vi "Actor Core.vi"(8 "error in":errorcluster, 11 "Hardware in":refnum<class "thorlabs_panel.lvclass">) -> (0 "error out":errorcluster, 3 "Actor out":refnum<class "Actor.lvclass">)   [LabVIEW 2015, in "thorlabs_panel.lvclass"]
doc: "(<B>Filename</B>: Actor Framework.lvlib:Actor.lvclass:Actor Core.vi)\n\nReceives messages to the actor, reacts to them, and initiates any error handling that may shut the actor down.\n\nDescendant classes may override this VI to append parallel tasks for the actor to complete while it handles messages. Overrides use the Call Parent Method node."
uses:
  thorlabs_panel.lvclass
  <vilib>/ActorFramework/Actor/Actor.lvclass
  UI/panel_class/panel.lvclass/panel.ctl
  <vilib>/ActorFramework/Actor/Actor.lvclass/Actor.ctl
  <vilib>/ActorFramework/Message Enqueuer/Message Enqueuer.lvclass/Message Enqueuer.ctl
  thorlabs_panel Messages/thorlabs_move_piezos Msg/thorlabs_move_piezos Msg.lvclass/thorlabs_move_piezos Msg.ctl
  thorlabs_panel Messages/thorlabs_connect Msg/thorlabs_connect Msg.lvclass/thorlabs_connect Msg.ctl
  <vilib>/ActorFramework/Message Enqueuer/Init from Existing Queue.vi
  <vilib>/ActorFramework/Message Enqueuer/Enqueue.vi
  <vilib>/ActorFramework/Message Priority Queue/Priority Enqueue.vi
  <vilib>/ActorFramework/Message Enqueuer/Message Enqueuer.lvclass
  thorlabs_panel Messages/thorlabs_move_piezos Msg/thorlabs_move_piezos Msg.lvclass
  thorlabs_panel Messages/thorlabs_zero_piezos Msg/thorlabs_zero_piezos Msg.lvclass
  thorlabs_panel Messages/thorlabs_connect Msg/thorlabs_connect Msg.lvclass
  thorlabs_panel Messages/thorlabs_query_positions Msg/thorlabs_query_positions Msg.lvclass
  UI/panel_class/panel.lvclass
panel:
  in  "step":dbl
  in  "right":bool
  in  "left":bool
  in  "down":bool
  in  "up":bool
  in  "zero_piezos":bool
  out "Z":dbl
  out "Y":dbl
  out "X":dbl
  in  "Speed":dbl
  in  "move_kinesis":bool
  in  "Z":dbl
  in  "Y":dbl
  in  "X":dbl
  out "Status":string
  in  "connect_kinesis":bool
  in  "Controller Serial":string="71827519"
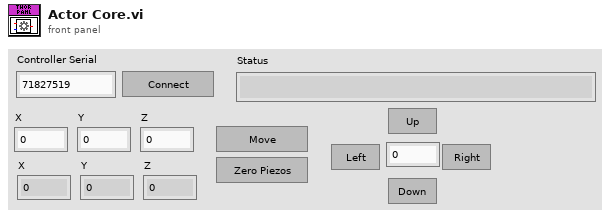
[diagram p1: front panel]
types:
  T1 = typedef "thorlabs_event_refs.ctl" = cluster{"Event Registration Refnum":refnum<event-registration>, "Event Registration Refnum":refnum<event-registration>}
  T2 = cluster{"Event Registration Refnum":refnum<event-registration>, "stop_ui_ref":refnum<event-registration>, "Event Registration Refnum":refnum<event-registration>}
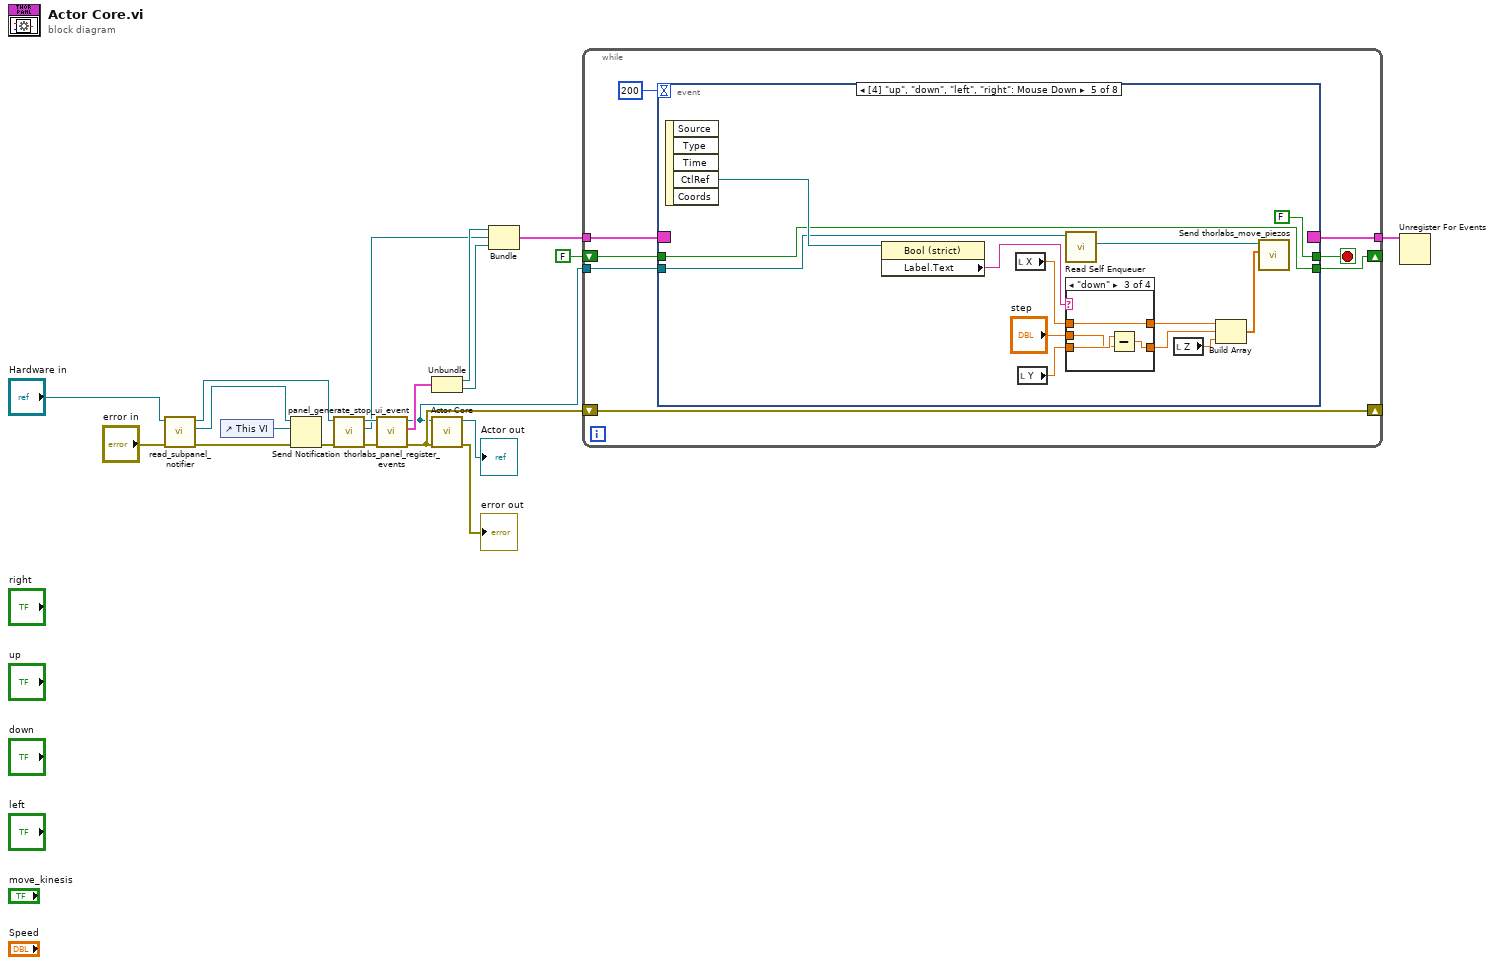
[diagram p0: block diagram]
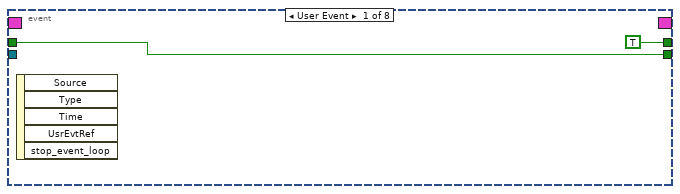
[diagram p2: hidden frame]
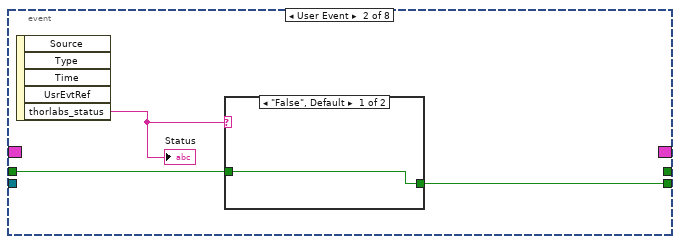
[diagram p3: hidden frame]
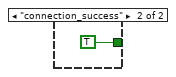
[diagram p4: hidden frame]
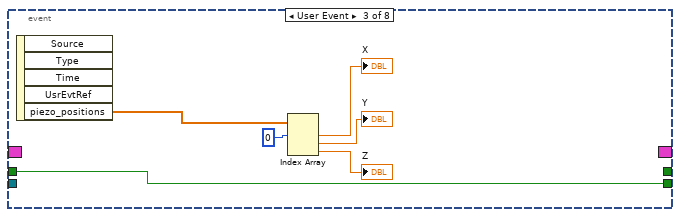
[diagram p5: hidden frame]
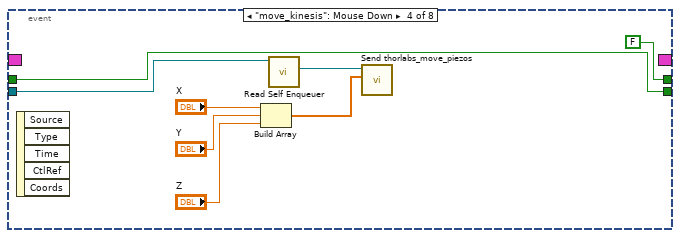
[diagram p6: hidden frame]
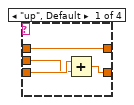
[diagram p7: hidden frame]
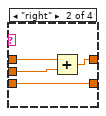
[diagram p8: hidden frame]
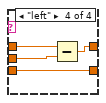
[diagram p9: hidden frame]
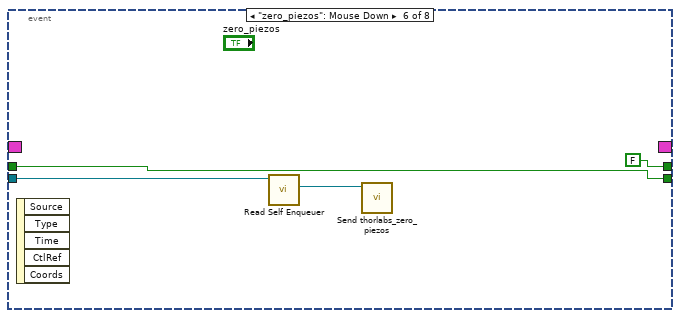
[diagram p10: hidden frame]
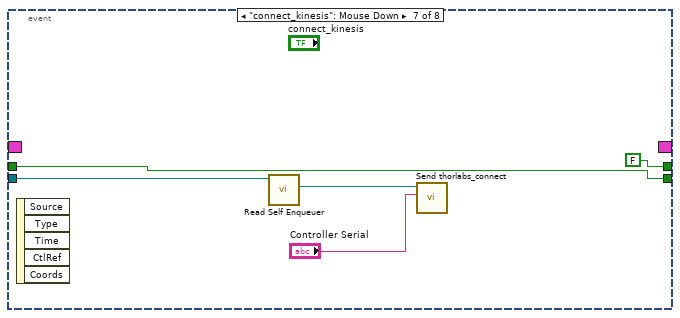
[diagram p11: hidden frame]
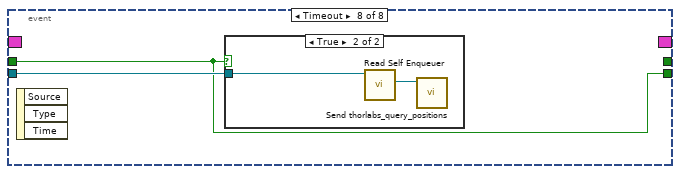
[diagram p12: hidden frame]
diagram:
  n1 = call "read_subpanel_notifier.vi"("error in (no error)"="error in", "panel in"="Hardware in") -> ("error out"=w14:errorcluster, "subpanel_notifier"=w16:refnum<notifier>, "panel out"=w15:refnum<class "thorlabs_panel.lvclass">)  [unwired: 7 in]
  n2 = control-ref of="This VI"() -> (w18:refnum<vi>)
  n3 = Send Notification(notification=w18, notifier=w16, error in (no error)=w14) -> (error out=w13:errorcluster)  [unwired: 1 out]
  n4 = call "panel_generate_stop_ui_event.vi"("error in (no error)"=w13, "panel in"=w15) -> ("error out"=w9:errorcluster, "stop_ui_ref"=w5:refnum<event-registration>, "panel out"=w10:refnum<class "thorlabs_panel.lvclass">)  [unwired: 7 in]
  n5 = call "thorlabs_panel_register_events.vi"("error in (no error)"=w9, "thorlabs_panel in"=w10) -> ("error out"=w8:errorcluster, "event_refs cluster"=w7:T1, "thorlabs_panel out"=w2:refnum<class "thorlabs_panel.lvclass">)  [unwired: 7 in]
  n6 = Unbundle(w7) -> ("Event Registration Refnum"=w6:refnum<event-registration>, "Event Registration Refnum"=w4:refnum<event-registration>)
  n7 = call-parent "Actor Core.vi"("error in"=w8, "Actor in"=w2) -> ("error out"=→"error out":errorcluster, "Actor out"=→"Actor out":refnum<class "Actor.lvclass">)  [unwired: 8 in]
  n8 = Bundle("Event Registration Refnum"=w6, "stop_ui_ref"=w5, "Event Registration Refnum"=w4) -> (w3:T2)  [unwired: 1 in]
  n9 = while {
    tunnel: w3 -> [w28]
    tunnel: [w26] -> w11
    shift-right: [w25] -> _
    shift-left: w8 -> [w25]
    tunnel: w2 -> [w24]
    shift-right: [w21] -> _
    shift-left: FALSE -> [w22]
    stop <- w27 stop-if-true
    n10 = event shown="[4] \"up\", \"down\", \"left\", \"right\": Mouse Down" {
      selector: w28 -> [_ _ _ _ _ _ _ _]
      dyn-events: [_ _ _ _ _ _ _ _] -> w26
      timeout: 200 -> [_ _ _ _ _ _ _ _]
      tunnel: [TRUE _ _ FALSE FALSE FALSE FALSE _] -> w27
      tunnel: w24 -> [_ _ _ w49 w52 w82 w87 w89]
      tunnel: w22 -> [w29 w32 w36 w42 w51 w80 w83 w88]
      tunnel: [w29 w31 w36 w42 w51 w80 w83 w88] -> w21
      event User Event {
        n11 = event-data() -> ()  [unwired: 1 in, 5 out]
      }
      event User Event {
        n12 = event-data() -> ("thorlabs_status"=w33:string)  [unwired: 1 in, 4 out]
        "Status" <- w33
        n13 = case shown="\"False\", Default" w33 {
          tunnel: w32 -> [w34 _]
          tunnel: [w34 TRUE] -> w31
          frame "False", Default {
          }
          frame "connection_success" {
          }
        }
      }
      event User Event {
        n14 = event-data() -> ("piezo_positions"=w41:dbl[])  [unwired: 1 in, 4 out]
        n15 = Index Array(array=w41, index #1=0 ("index")) -> (element #1=→"X":dbl, element #2=→"Y":dbl, element #3=→"Z":dbl)  [unwired: 2 in]
      }
      event "move_kinesis": Mouse Down {
        n16 = event-data() -> ()  [unwired: 1 in, 5 out]
        n17 = Build Array("X", "Y", "Z") -> (w44:dbl[])
        n18 = call <vilib>:"Read Self Enqueuer.vi"("Actor"=w49) -> ("Self Enqueuer"=w43:refnum<class "Message Enqueuer.lvclass">)  [unwired: 10 in]
        n19 = call "Send thorlabs_move_piezos.vi"("new_positions"=w44, "Message Enqueuer"=w43) -> ()  [unwired: 8 in, 2 out]
      }
      event "up", "down", "left", "right": Mouse Down {
        n20 = event-data() -> ("CtlRef"=w62:refnum<vi>)  [unwired: 1 in, 4 out]
        n21 = property class="Bool (strict)"(reference=w62) -> ("Label.Text"=w61:string)  [unwired: 1 in, 2 out]
        n22 = local read "X"() -> (w56:dbl)
        n23 = local read "Y"() -> (w59:dbl)
        n24 = call <vilib>:"Read Self Enqueuer.vi"("Actor"=w52) -> ("Self Enqueuer"=w53:refnum<class "Message Enqueuer.lvclass">)  [unwired: 10 in]
        n25 = case shown="\"down\"" w61 {
          tunnel: w59 -> [w66 w67 w74 w75]
          tunnel: "step" -> [w65 w70 w73 w78]
          tunnel: [w64 w67 w72 w75] -> w57
          tunnel: w56 -> [w63 w69 w71 w77]
          tunnel: [w63 w68 w71 w76] -> w55
          frame "up", Default {
            n26 = Add(x=w66, y=w65) -> (x+y=w64:dbl)
          }
          frame "right" {
            n27 = Add(x=w69, y=w70) -> (x+y=w68:dbl)
          }
          frame "down" {
            n28 = Subtract(x=w74, y=w73) -> (x-y=w72:dbl)
          }
          frame "left" {
            n29 = Subtract(x=w77, y=w78) -> (x-y=w76:dbl)
          }
        }
        n30 = local read "Z"() -> (w60:dbl)
        n31 = Build Array(w55, w57, w60) -> (w54:dbl[])
        n32 = call "Send thorlabs_move_piezos.vi"("new_positions"=w54, "Message Enqueuer"=w53) -> ()  [unwired: 8 in, 2 out]
      }
      event "zero_piezos": Mouse Down {
        n33 = event-data() -> ()  [unwired: 1 in, 5 out]
        n34 = call <vilib>:"Read Self Enqueuer.vi"("Actor"=w82) -> ("Self Enqueuer"=w81:refnum<class "Message Enqueuer.lvclass">)  [unwired: 10 in]
        n35 = call "Send thorlabs_zero_piezos.vi"("Message Enqueuer"=w81) -> ()  [unwired: 9 in, 2 out]
      }
      event "connect_kinesis": Mouse Down {
        n36 = event-data() -> ()  [unwired: 1 in, 5 out]
        n37 = call <vilib>:"Read Self Enqueuer.vi"("Actor"=w87) -> ("Self Enqueuer"=w86:refnum<class "Message Enqueuer.lvclass">)  [unwired: 10 in]
        n38 = call "Send thorlabs_connect.vi"("Serial"="Controller Serial", "Message Enqueuer"=w86) -> ()  [unwired: 8 in, 2 out]
      }
      event Timeout {
        n39 = event-data() -> ()  [unwired: 1 in, 3 out]
        n40 = case shown="True" w88 {
          tunnel: w89 -> [_ w91]
          frame False {
          }
          frame True {
            n41 = call <vilib>:"Read Self Enqueuer.vi"("Actor"=w91) -> ("Self Enqueuer"=w90:refnum<class "Message Enqueuer.lvclass">)  [unwired: 10 in]
            n42 = call "Send thorlabs_query_positions.vi"("Message Enqueuer"=w90) -> ()  [unwired: 9 in, 2 out]
          }
        }
      }
    }
  }
  n43 = Unregister For Events(event registration refnum=w11) -> ()  [unwired: 1 in, 1 out]
